vi "VariableScan.vi"(1 "Scan-to-GUI":T1, 2 "GUI-to-Scan":T1) -> ()   [LabVIEW 2018]
uses:
  VariableScan_Cluster.ctl
  <vilib>/NI/AMC/Message Queue.ctl
  <vilib>/NI/AMC/Message.ctl
  <vilib>/NI/Tools/Keyed Array/KeyedArray.ctl
  <vilib>/NI/AMC/Read Termination Message.vi
  <vilib>/NI/AMC/Create Single Message.vi
  <vilib>/NI/AMC/Update Message Routing Info.vi
  <vilib>/NI/AMC/Globals.vi
  <vilib>/NI/AMC/Send Message.vi
  <vilib>/NI/AMC/AMC.lvlib
  <vilib>/NI/Tools/Keyed Array/Tools_KeyedArray.lvlib
panel:
  in  "stop":bool
  in  "Variable Cluster":T2={"Values"=[0.10000000000000003, 0.20000000000000004, 0.30000000000000004], "Action"=1, "Inst."=0, "# Elements"=3, "Next Element"=0, "First Val"=0.10000000000000003, "Final Val"=0.30000000000000004, "Update Array"=FALSE, "Description"="", "Variable Type"=0, "Scan Now"=FALSE, "# Act/Inst."=2, "Electrodes_range"=[], "Parameter Name"="RW&f_start (Hz)", "# Passes"=1} {"Variable Type" items=["Duration (s)", "Voltage (V)", "Parameter", "Repetitions"]; "Final Val" format="%_6p"; "First Val" format="%_6p"; "Values" format="%_6p"}
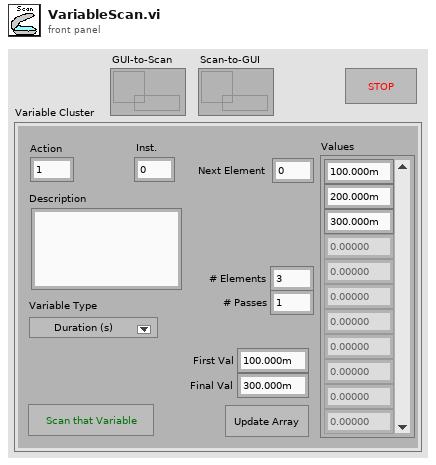
[diagram p1: front panel]
types:
  T1 = typedef "AMC.lvlib/Message Queue.ctl" = refnum<queue>
  T2 = typedef "VariableScan_Cluster.ctl" = cluster{"Values":dbl[], "Action":i32, "Inst.":i32, "# Elements":i32, "Next Element":i32, "First Val":dbl, "Final Val":dbl, "Update Array":bool, "Description":string, "Variable Type":u16, "Scan Now":bool, "# Act/Inst.":i32, "Electrodes_range":i32[], "Parameter Name":string, "# Passes":i32}
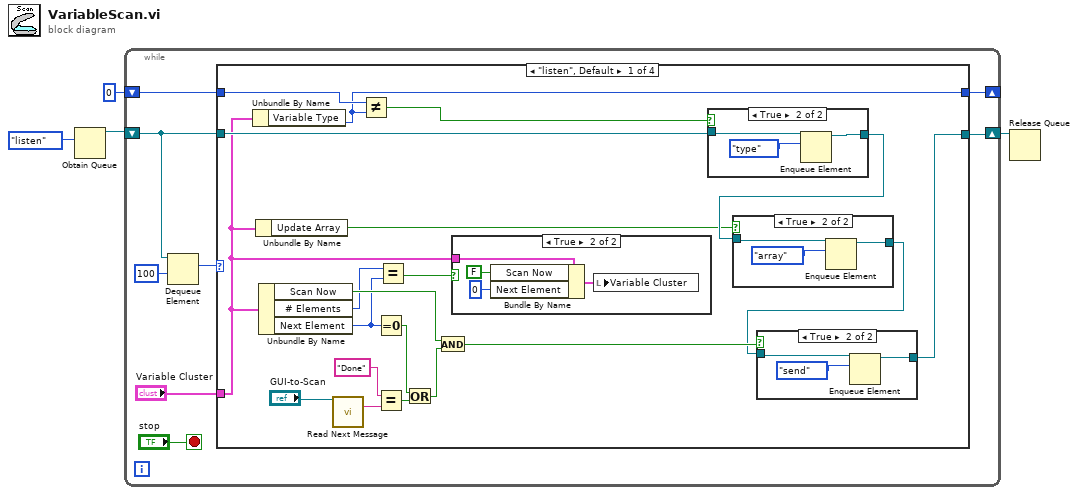
[diagram p0: block diagram]
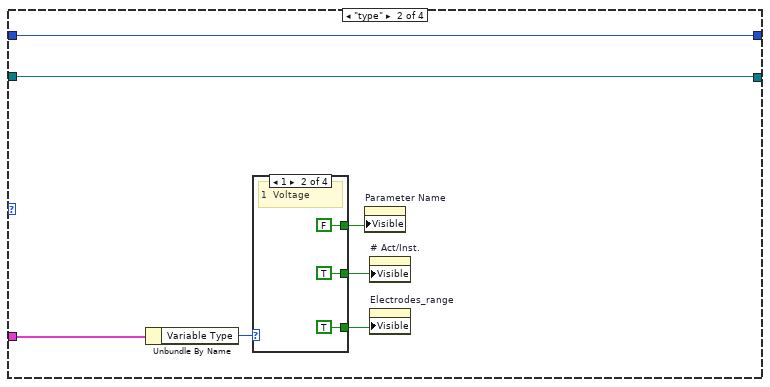
[diagram p6: hidden frame]
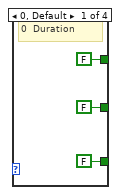
[diagram p7: hidden frame]
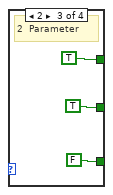
[diagram p8: hidden frame]
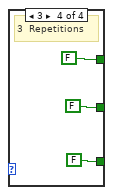
[diagram p9: hidden frame]
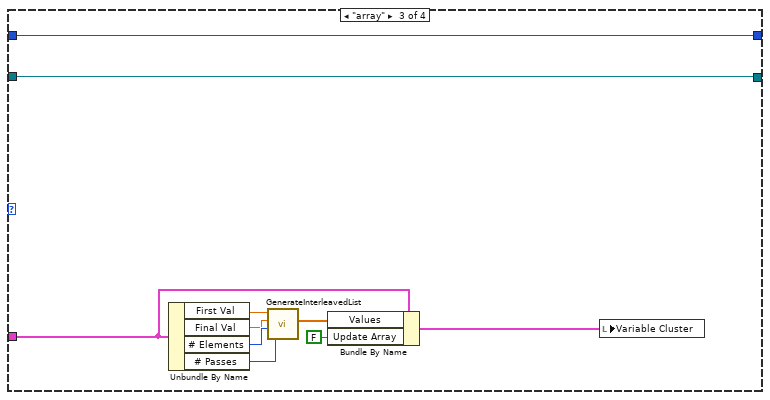
[diagram p10: hidden frame]
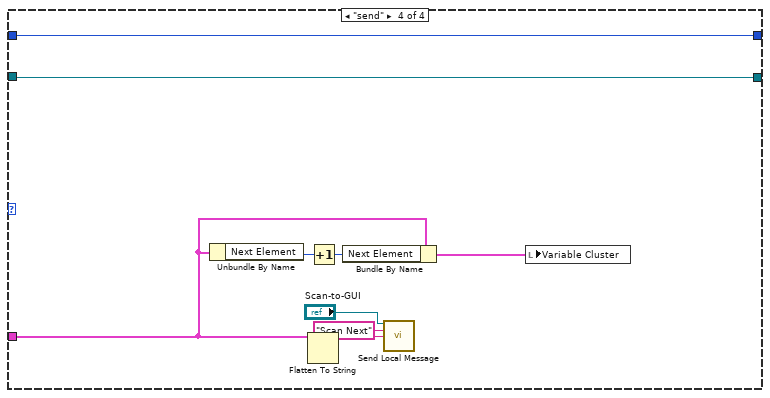
[diagram p11: hidden frame]
diagram:
  n1 = Obtain Queue(element data type=enum16{"listen", "type", "array", "send"}."listen" ("mode")) -> (queue out=w4:refnum<queue>)  [unwired: 4 in, 2 out]
  n2 = while {
    shift-right: [w9] -> _
    shift-left: u16 0 ("Variable Type") -> [w10]
    shift-right: [w8] -> w1
    shift-left: w4 -> [w7]
    stop <- "stop" stop-if-true
    n3 = Dequeue Element(queue=w7, timeout in ms (-1)=100) -> (element=w6:enum16{"listen", "type", "array", "send"})  [unwired: 1 in, 3 out]
    n4 = case shown="\"listen\", Default" w6 {
      tunnel: "Variable Cluster" -> [w16 w52 w70 w79]
      tunnel: w10 -> [w31 w49 w69 w86]
      tunnel: [w30 w49 w69 w86] -> w9
      tunnel: [w20 w50 w68 w85] -> w8
      tunnel: w7 -> [w28 w50 w68 w85]
      frame "listen", Default {
        n5 = Unbundle By Name(w16) -> ("Variable Type"=w30:u16)
        n6 = Unbundle By Name(w16) -> ("Update Array"=w15:bool)
        n7 = Unbundle By Name(w16) -> ("Scan Now"=w23:bool, "# Elements"=w18:i32, "Next Element"=w19:i32)
        n8 = call <vilib>:"Read Next Message.vi"("message queue in"="GUI-to-Scan") -> ("message name"=w13:string)  [unwired: 7 in, 7 out]
        n9 = Not Equal?(x=w31, y=w30) -> (x != y?=w29:bool)
        n10 = Equal To 0?(x=w19) -> (x = 0?=w25:bool)
        n11 = Equal?(x="Done", y=w13) -> (x = y?=w26:bool)
        n12 = Equal?(x=w18, y=w19) -> (x = y?=w17:bool)
        n13 = Or(x=w25, y=w26) -> (x .or. y?=w24:bool)
        n14 = And(x=w23, y=w24) -> (x .and. y?=w27:bool)
        n15 = case shown="True" w17 {
          tunnel: w16 -> [_ w36]
          frame False {
          }
          frame True {
            n16 = Bundle By Name(cluster=w36, "Scan Now"=FALSE, "Next Element"=0) -> (w33:T2)
            n17 = local write "Variable Cluster"(w33) -> ()
          }
        }
        n18 = case shown="True" w29 {
          tunnel: w28 -> [w45 w47]
          tunnel: [w45 w46] -> w21
          frame False {
          }
          frame True {
            n19 = Enqueue Element(queue=w47, element=enum16{"listen", "type", "array", "send"}."type" ("mode")) -> (queue out=w46:refnum<queue>)  [unwired: 2 in, 2 out]
          }
        }
        n20 = case shown="True" w15 {
          tunnel: w21 -> [w37 w39]
          tunnel: [w37 w38] -> w22
          frame False {
          }
          frame True {
            n21 = Enqueue Element(queue=w39, element=enum16{"listen", "type", "array", "send"}."array" ("mode")) -> (queue out=w38:refnum<queue>)  [unwired: 2 in, 2 out]
          }
        }
        n22 = case shown="True" w27 {
          tunnel: w22 -> [w41 w43]
          tunnel: [w41 w42] -> w20
          frame False {
          }
          frame True {
            n23 = Enqueue Element(queue=w43, element=enum16{"listen", "type", "array", "send"}."send" ("mode")) -> (queue out=w42:refnum<queue>)  [unwired: 2 in, 2 out]
          }
        }
      }
      frame "type" {
        n24 = Unbundle By Name(w52) -> ("Variable Type"=w51:u16)
        n25 = case shown="1" w51 {
          tunnel: [FALSE ("Visible") TRUE ("Visible") FALSE ("Visible") FALSE ("Visible")] -> w53
          tunnel: [FALSE ("Visible") TRUE ("Visible") TRUE ("Visible") FALSE ("Visible")] -> w54
          tunnel: [FALSE ("Visible") FALSE ("Visible") TRUE ("Visible") FALSE ("Visible")] -> w55
          frame 0, Default {
            # "0  Duration"
          }
          frame 1 {
            # "1  Voltage"
          }
          frame 2 {
            # "2  Parameter"
          }
          frame 3 {
            # "3  Repetitions"
          }
        }
        n26 = property on="Parameter Name" class="Str"("Visible"=w55) -> ()  [unwired: 2 in, 2 out]
        n27 = property on="# Act/Inst." class="DigNum (strict)"("Visible"=w54) -> ()  [unwired: 2 in, 2 out]
        n28 = property on="Electrodes_range" class="Arr (strict)"("Visible"=w53) -> ()  [unwired: 2 in, 2 out]
      }
      frame "array" {
        n29 = Unbundle By Name(w70) -> ("First Val"=w73:dbl, "Final Val"=w74:dbl, "# Elements"=w75:i32, "# Passes"=w76:i32)
        n30 = call "GenerateInterleavedList.vi"("# passes"=w76, "# points"=w75, "Stop"=w74, "Start"=w73) -> ("Array"=w77:dbl[])  [unwired: 2 in, 1 out]
        n31 = Bundle By Name(cluster=w70, "Values"=w77, "Update Array"=FALSE) -> (w72:T2)
        n32 = local write "Variable Cluster"(w72) -> ()
      }
      frame "send" {
        n33 = Unbundle By Name(w79) -> ("Next Element"=w82:i32)
        n34 = Flatten To String(anything=w79) -> (data string=w81:string)  [unwired: 3 in, 2 out]
        n35 = Increment(x=w82) -> (x+1=w83:i32)
        n36 = Bundle By Name(cluster=w79, "Next Element"=w83) -> (w84:T2)
        n37 = call <vilib>:"Send Local Message.vi"("message queue in"="Scan-to-GUI", "message name"="Scan Next", "message value"=w81) -> ()  [unwired: 10 in, 3 out]
        n38 = local write "Variable Cluster"(w84) -> ()
      }
    }
  }
  n39 = Release Queue(queue=w1) -> ()  [unwired: 2 in, 3 out]
